vi "Get UI Details.vi"(8 "error in":errorcluster) -> (0 "error out":errorcluster, 3 "user_interface_details":T1)   [LabVIEW 2020, in "MeasurementService_Template.lvlib" / "MeasurementService_Template.lvclass"]
uses:
  MeasurementService_Template.lvclass
  RPC Messages/Measurement_v1_UserInterfaceDetails/Measurement_v1_UserInterfaceDetails_Data.ctl
  Measurement UI.vi
  MeasurementService_Template.lvlib
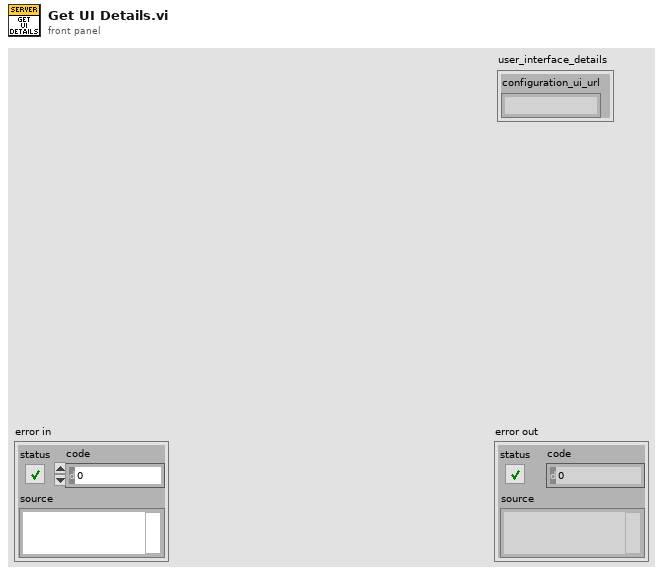
[diagram p1: front panel]
types:
  T1 = typedef "MeasurementService_Template.lvlib/MeasurementService_Template.lvclass/Measurement_v1_UserInterfaceDetails_Data.ctl" = cluster{"configuration_ui_url":string}
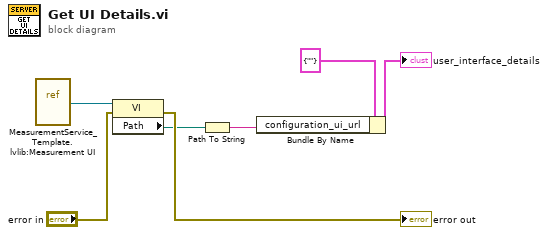
[diagram p0: block diagram]
diagram:
  n1 = vi-ref "MeasurementService_Template.lvlib:Measurement UI.vi"() -> (w5:refnum<vi>)
  n2 = property class="VI"(reference=w5, error in="error in") -> (error out=→"error out":errorcluster, "Path"=w2:path)  [unwired: 1 out]
  n3 = Path To String(path=w2) -> (string=w1:string)
  n4 = Bundle By Name(cluster=T1 {"configuration_ui_url"=""} ("user_interface_details"), "configuration_ui_url"=w1) -> (→"user_interface_details":T1)
